vi "Test Euler Angle Conversion.vi"() -> ()   [LabVIEW 2023]
uses:
  Orient3d.lvclass
panel:
  out "phi/roll":dbl format="%#.3f"
  out "theta/pitch":dbl format="%#.3f"
  out "psi/yaw":dbl format="%#.3f"
  in  "phi/roll":dbl
  in  "theta/pitch":dbl
  in  "psi/yaw":dbl
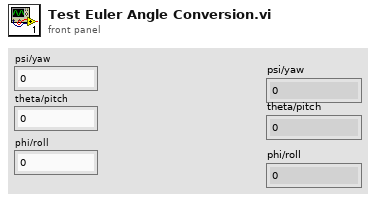
[diagram p1: front panel]
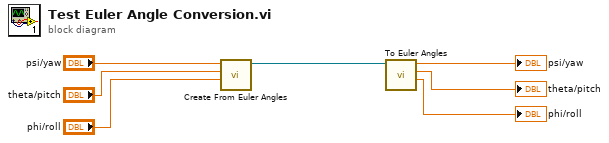
[diagram p0: block diagram]
diagram:
  n1 = call "Create From Euler Angles.vi"("phi/roll"="phi/roll", "theta/pitch"="theta/pitch", "psi/yaw"="psi/yaw") -> ("Orient3d out"=w4:refnum<class "Orient3d.lvclass">)  [unwired: 7 in, 1 out]
  n2 = call "To Euler Angles.vi"("Orient3d in"=w4) -> ("phi/roll"=→"phi/roll":dbl, "theta/pitch"=→"theta/pitch":dbl, "psi/yaw"=→"psi/yaw":dbl)  [unwired: 7 in, 1 out]
